vi "Error Converter (ErrCode or Status).vi"(8 "error in (no error)":errorcluster caption="错误输入（无错误）", 11 "error code":i32 caption="错误代码") -> (0 "error out":errorcluster caption="错误输出")   [LabVIEW 2020]
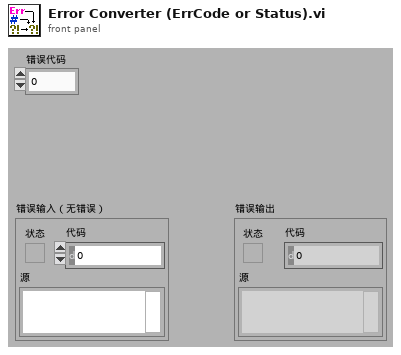
[diagram p1: front panel]
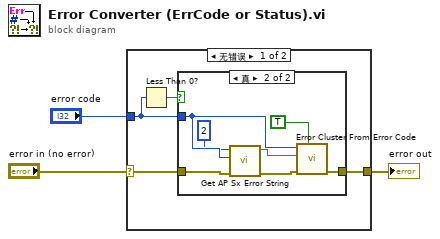
[diagram p0: block diagram]
diagram:
  n1 = case shown="无错误" "error in (no error)" {
    selector: "error in (no error)" -> [w6 w16]
    tunnel: [w4 w16] -> w2
    tunnel: "error code" -> [w5 _]
    frame No Error {
      n2 = Less Than 0?(x=w5) -> (x < 0?=w7:bool)
      n3 = case shown="真" w7 {
        tunnel: w6 -> [w8 w13]
        tunnel: w5 -> [_ w12]
        tunnel: [w8 w15] -> w4
        frame False {
        }
        frame True {
          n4 = call "Get AP Sx Error String.vi"("error in (no error)"=w13, "error"=w12, "pgiType"=2) -> ("error out"=w10:errorcluster, "function return"=w9:string)  [unwired: 7 in]
          n5 = call <vilib>:"Error Cluster From Error Code.vi"("show call chain? (False)"=TRUE, "error in (no error)"=w10, "error message (\"\")"=w9, "error code (0)"=w12) -> ("error out"=w15:errorcluster)  [unwired: 5 in]
        }
      }
    }
    frame Error {
    }
  }
  "error out" <- w2
